vi "serial_01.vi"(0 "VISA resource name":refnum<visa-resource-name>="COM5") -> ()   [LabVIEW 2010]
doc: "The Basic Serial Read and Write example performs a Serial Port Read, a Serial Port Write, or a combination of these actions. The user selects the actions (read or write) on the front panel. If both are selected, the VI will write the data first, read data, and then close the VISA session that is opened to the port. This VI will wait until the specified number of bytes is received at the port. Only the number of bytes specified will be read.\n\nINSTRUCTIONS:\n1) Select the serial resource and configuration parameters (baud rate, data bits, parity, stop bits, flow control).\n2) Select the operations to be performed. \n3) Connect the serial port to your device. If no device is available, perform a loopback test by doing one of the following. Short pins 2 and 3 on a RS-232 cable or short pin 4 to pin 8 and pin 5 to pin 9 on a RS-485/422 cable. \n4) Run the VI to see the data read. (The \"read string\" will match the \"string to write\" if a loopback test was performed.)\n\nNote: The parameters set for the serial port must match the parameters of the connected instrument or device. In this example, the bytes to read parameter specifies the number of bytes that the serial port reads. If there were more bytes at the port than the number specified in bytes to read, those bytes would not be read. Also, if you specify to read more bytes than the number of bytes actually read, you might receive a timeout error message.\n\nOn the block diagram, the Configure Serial Port VI sets the configuration parameters. The front panel displays the controls used to configure the basic parameters, such as baud rate, data bits, and parity. Constants configure the other parameters the user probably does not need set. After the VISA Configure Serial Port VI opens the VISA session and configures the port, the VI passes the VISA resource name to other VIs that perform operations on that VISA resource. The VISA Write function sends a command to the serial device and the VISA Read function returns data based on the command. The VISA Close function then closes the reference to the serial device. It is important to close the reference; otherwise communication through with that port through protocols other than VISA might not be possible."
uses:
  <vilib>/Instr/_visa.llb/VISA Configure Serial Port (Instr).vi
panel:
  in  "Start":bool=TRUE
  out "Meter":dbl(knob)=668.0 scale=0.0..1024.0
  out "Afisare grafica intrare analogica A0":i32(graph)=668
  # "Stop"
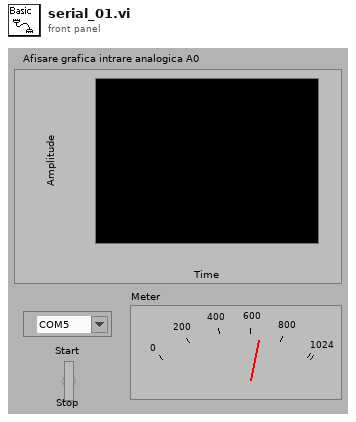
[diagram p1: front panel]
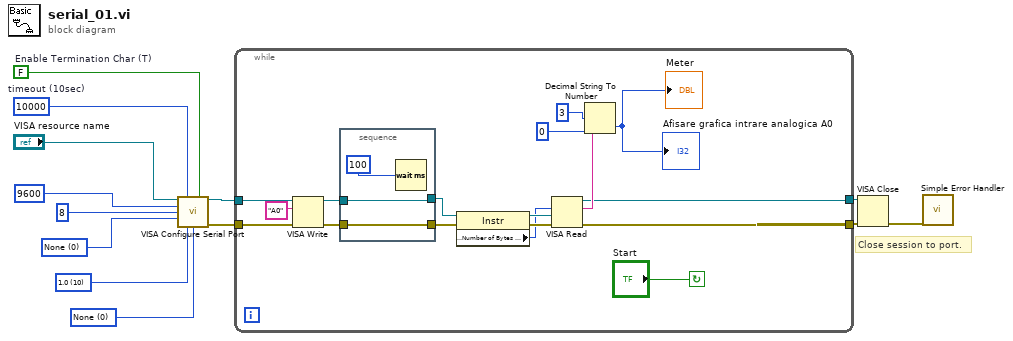
[diagram p0: block diagram]
diagram:
  w6 = u16 0 items=["None", "Odd", "Even", "Mark", "Space"] ("parity")
  w3 = u16 10 items=["1.0"=10, "1.5"=15, "2.0"=20] ("stop bits")
  w2 = u16 0 items=["None"=0, "XON/XOFF"=1, "RTS/CTS"=2, "DTR/DSR"=4] ("flow control")
  w4 = FALSE  # Enable Termination Char (T)
  w5 = u32 10000  # timeout (10sec)
  # "Close session to port."
  n1 = call-poly "VISA Configure Serial Port"("VISA resource name"="VISA resource name", "timeout (10sec)"=w5, "Enable Termination\nChar (T)"=w4, "baud rate (9600)"=u32 9600 ("baud rate"), "data bits (8)"=u16 8 ("data bits"), "parity (0:none)"=w6, "stop bits (10: 1 bit)"=w3, "flow control (0:none)"=w2) -> ("VISA resource name out"=w10:refnum<visa-resource-name>, "error out"=w11:errorcluster)  [unwired: 1 in, 5 out]
  n2 = while {
    tunnel: w11 -> [w27]
    tunnel: w10 -> [w28]
    tunnel: [w16] -> w9
    tunnel: [w17] -> w8
    stop <- "Start" continue-if-true
    n3 = VISA Write(VISA resource name=w28, write buffer="A0" ("string to write"), error in (no error)=w27) -> (VISA resource name out=w26:refnum<visa-resource-name>, error out=w25:errorcluster)  [unwired: 1 out]
    n4 = stacked-sequence {
      tunnel: w26 -> [w32]
      tunnel: w25 -> [w31]
      tunnel: [w32] -> w15
      tunnel: [w31] -> w14
      frame #0 {
        n5 = Wait (ms)(milliseconds to wait=u32 100 ("delay before read (ms)")) -> ()  [unwired: 1 out]
      }
    }
    n6 = property class="Instr"(reference=w15, error in=w14) -> (reference out=w24:refnum<visa-resource-name>, error out=w23:errorcluster, "Serial Settings:Number of Bytes at Serial Port"=w22:u32)
    n7 = VISA Read(VISA resource name=w24, byte count=w22, error in (no error)=w23) -> (VISA resource name out=w17:refnum<visa-resource-name>, read buffer=w21:string, error out=w16:errorcluster)  [unwired: 1 out]
    n8 = Decimal String To Number(string=w21, offset=3, default (0L)=0) -> (number=→"Afisare grafica intrare analogica A0" →"Meter":i32)  [unwired: 1 out]
  }
  n9 = VISA Close(VISA resource name=w8, error in (no error)=w9) -> (error out=w7:errorcluster)
  n10 = call <vilib>:"Simple Error Handler.vi"("error in (no error)"=w7) -> ()  [unwired: 1 in, 8 out]
